vi "blowfish_encipher.vi"(8 "error in (no error)":errorcluster, 11 "Input Text":string) -> (0 "error out":errorcluster, 3 "Output Text":string)   [LabVIEW 2020]
doc: "The Blowfish Encryption Algorithm\n\nBlock cipher: 64-bit block \nVariable key length: 32 bits to 448 bits \nDesigned by Bruce Schneier \nMuch faster than DES and IDEA \nUnpatented and royalty-free \nNo license required \n\nBlowfish is a symmetric block cipher that can be used as a drop-in replacement for DES or IDEA. It takes a variable-length key, from 32 bits to 448 bits, making it ideal for both domestic and exportable use. Blowfish was designed in 1993 by Bruce Schneier as a fast, free alternative to existing encryption algorithms. Since then it has been analyzed considerably, and it is slowly gaining acceptance as a strong encryption algorithm. Blowfish is unpatented and license-free, and is available free for all uses.\n\nAs far as I know this is the first implementation of the Blowfish Algorithm in LabVIEW. With this set of subvi's one can encrypt data in LabVIEW without the need of external software. This can be used to send data securely over Data socket as well as TCP and UDP communications. And also protect remote control systems from unauthorized access, by encrypting the control communications.\n\nI welcome any constructive commits, and bug reports can be sent to the E-mail contained in the code"
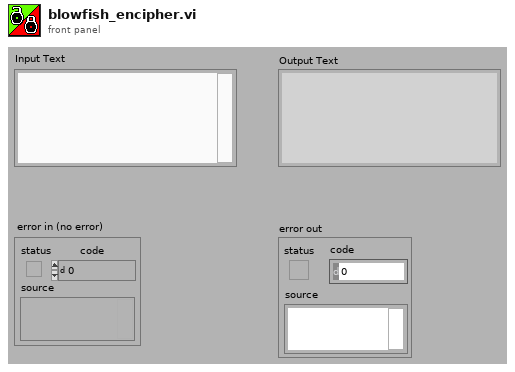
[diagram p1: front panel]
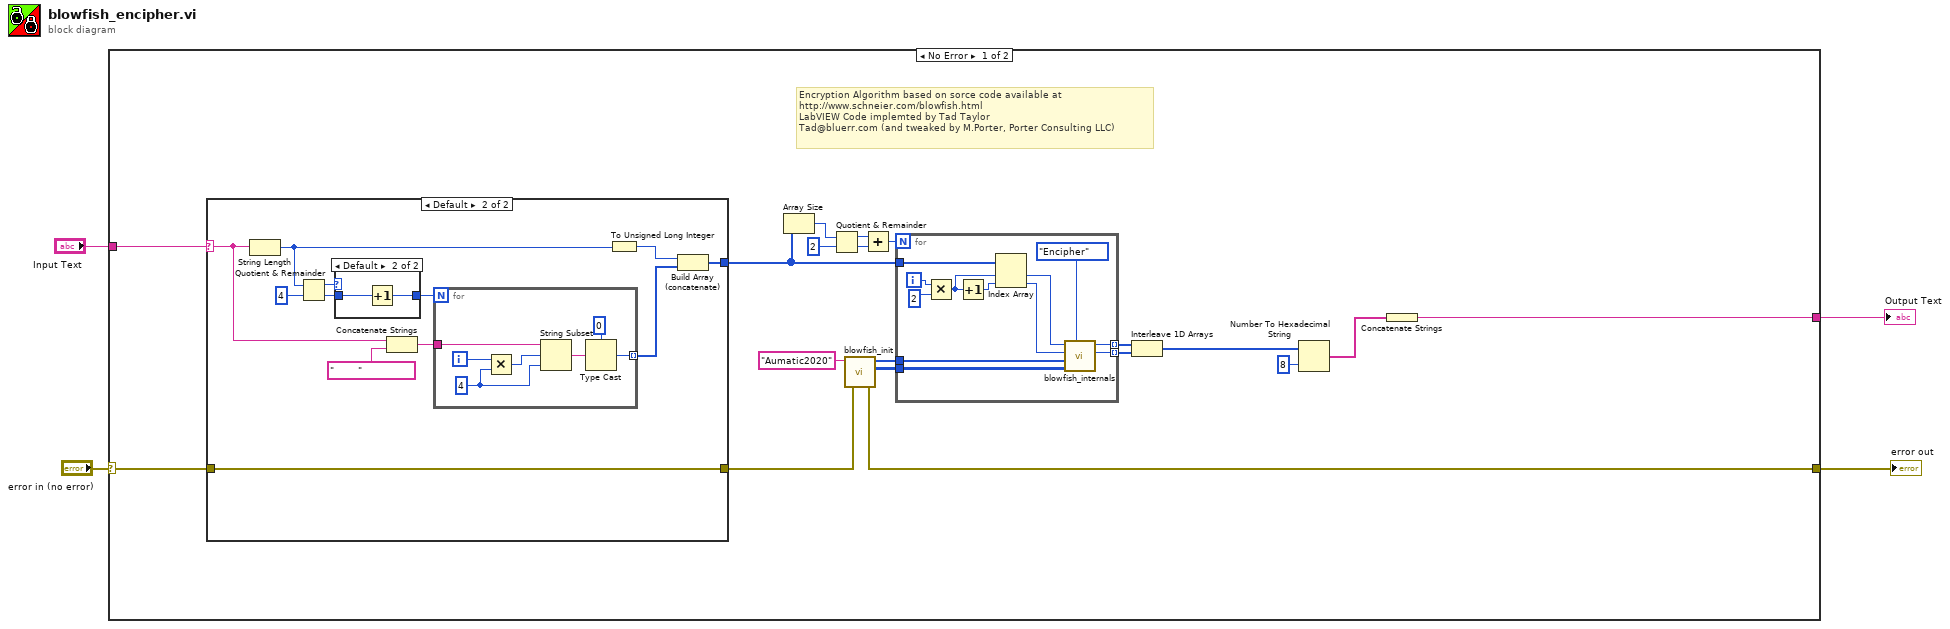
[diagram p0: block diagram]
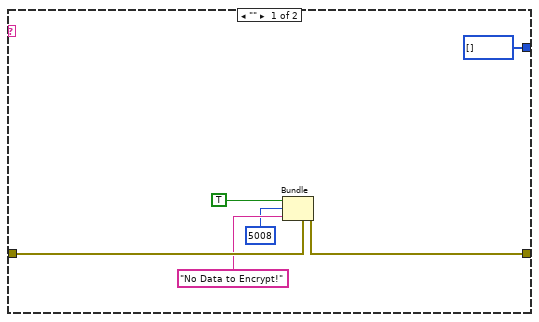
[diagram p2: hidden frame]
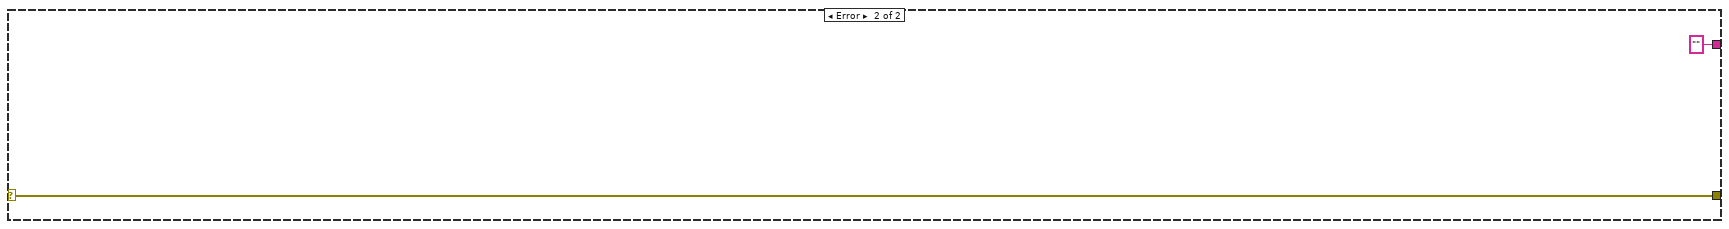
[diagram p4: hidden frame]
diagram:
  n1 = case shown="No Error" "error in (no error)" {
    selector: "error in (no error)" -> [w16 w64]
    tunnel: [w10 "" ("data string")] -> w3
    tunnel: [w9 w64] -> w2
    tunnel: "Input Text" -> [w5 _]
    frame No Error {
      # "Encryption Algorithm based on sorce code available at\nhttp://www.schneier.com/blowfish.html\nLabVIEW Code implemted by Tad Taylor\nTad@bluerr.com (and tweaked by M.Porter, Porter Consulting LLC)"
      n2 = case shown="Default" w5 {
        selector: w5 -> [_ w31]
        tunnel: [u32[] [] w35] -> w18
        tunnel: w16 -> [w28 w30]
        tunnel: [w27 w30] -> w17
        frame "" {
          n3 = Bundle(cluster=w28, "status"=TRUE ("Halt?"), "code"=5008 ("Halt Code"), "source"="No Data to Encrypt!" ("Halt Message")) -> (w27:errorcluster)
        }
        frame Default {
          n4 = String Length(string=w31) -> (length=w37:i32)
          n5 = Quotient & Remainder(x=w37, y=4) -> (x-y*floor(x/y)=w34:i32, floor(x/y)=w33:i32)
          n6 = case shown="Default" w34 {
            tunnel: w33 -> [w42 w44]
            tunnel: [w42 w43] -> w32
            frame 0 {
            }
            frame Default {
              n7 = Increment(x=w44) -> (x+1=w43:i32)
            }
          }
          n8 = Concatenate Strings(w31, "        ") -> (w38:string)
          n9 = for {
            N: w32 -> [_]
            tunnel: w38 -> [w49]
            tunnel: [w50] -> w40 mode=indexing
            i -> [w47]
            w45 = 4 ("length (rest)")
            n10 = Multiply(x=w47, y=w45) -> (x*y=w46:i32)
            n11 = String Subset(string=w49, offset (0)=w46, length (rest)=w45) -> (substring=w48:string)
            n12 = Type Cast(type=u32 0, x=w48) -> (*(type *) &x=w50:u32)
          }
          n13 = To Unsigned Long Integer(number=w37) -> (unsigned 32bit integer=w41:u32)
          n14 = Build Array (concatenate)(w41, w40) -> (w35:u32[])
        }
      }
      n15 = Array Size(array=w18) -> (size(s)=w15:i32)
      n16 = Quotient & Remainder(x=w15, y=2 ("x")) -> (x-y*floor(x/y)=w11:i32, floor(x/y)=w12:i32)
      n17 = call "blowfish_init.vi"("error in (no error)"=w17, "Key"="Aumatic2020") -> ("error out"=w9:errorcluster, "S 4X256"=w22:u32[][], "P 18"=w23:u32[])  [unwired: 3 in]
      n18 = Add(x=w11, y=w12) -> (x+y=w13:i32)
      n19 = for {
        N: w13 -> [_]
        tunnel: [w55] -> w21 mode=indexing
        tunnel: [w54] -> w20 mode=indexing
        tunnel: w23 -> [w58]
        tunnel: w22 -> [w59]
        tunnel: w18 -> [w63]
        i -> [w62]
        n20 = Multiply(x=w62, y=2 ("element")) -> (x*y=w61:i32)
        n21 = Increment(x=w61) -> (x+1=w53:i32)
        n22 = Index Array(array=w63, index #1=w61, index #2=w53) -> (element #1=w57:u32, element #2=w56:u32)
        n23 = call "blowfish_internals.vi"("Enc/Dec"=enum16{"Encipher", "Decipher"}."Encipher", "S 4X256"=w59, "P 18"=w58, "Xr"=w56, "Xl"=w57) -> ("Xr out"=w54:u32, "Xl out"=w55:u32)  [unwired: 2 in]
      }
      n24 = Interleave 1D Arrays(w21, w20) -> (w19:u32[])
      n25 = Number To Hexadecimal String(1:i16 8 ("width (-)"), 2:w19) -> (0:w6:string[])
      n26 = Concatenate Strings(w6) -> (w10:string)
    }
    frame Error {
    }
  }
  "error out" <- w2
  "Output Text" <- w3
